vi "Tray_SetTray.vi"(7 "Initial color":u32(colorbox)=16448250, 8 "error in (no error)":errorcluster, 9 "GridSize":cluster{"x":u32, "y":u32}, 10 "MaxArea":cluster{"x":u32, "y":u32}, 11 "Tray in":refnum<vi>) -> (0 "error out":errorcluster)   [LabVIEW 2019]
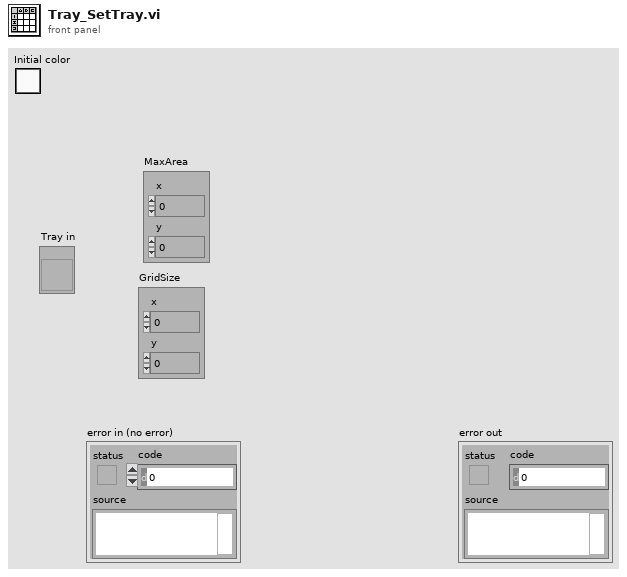
[diagram p1: front panel]
types:
  T1 = typedef "LVPositionTypeDef.ctl" = cluster{"Left":i32, "Top":i32}
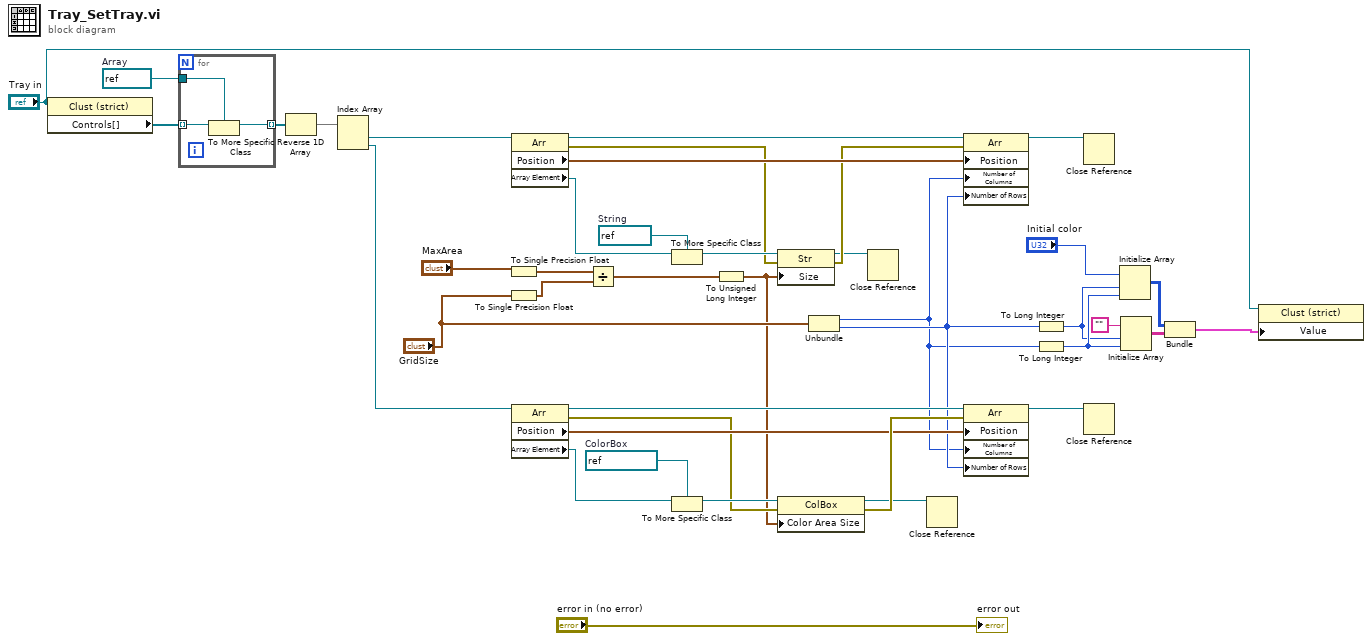
[diagram p0: block diagram]
diagram:
  w17 = refnum<vi> refnum  # Array
  w41 = refnum<vi> refnum  # String
  w38 = refnum<vi> refnum  # ColorBox
  n1 = property class="Clust (strict)"(reference="Tray in") -> ("Controls[]"=w18:refnum<vi>[])  [unwired: 1 in, 2 out]
  n2 = for {
    tunnel: w18 -> [w44] mode=indexing
    tunnel: w17 -> [w43]
    tunnel: [w42] -> w16 mode=indexing
    n3 = To More Specific Class(target class=w43, reference=w44) -> (specific class reference=w42:refnum<vi>)  [unwired: 1 in, 1 out]
  }
  n4 = Reverse 1D Array(array=w16) -> (reversed array=w15:refnum<vi>[])
  n5 = Index Array(array=w15) -> (element #1=w14:refnum<vi>, element #2=w13:refnum<vi>)  [unwired: 2 in]
  n6 = To Single Precision Float(number="MaxArea") -> (single precision float=w12:cluster{"x":sgl, "y":sgl})
  n7 = To Single Precision Float(number="GridSize") -> (single precision float=w10:cluster{"x":sgl, "y":sgl})
  n8 = property class="Arr"(reference=w14) -> (reference out=w32:refnum<vi>, error out=w33:errorcluster, "Position"=w35:T1, "Array Element"=w39:refnum<vi>)  [unwired: 1 in]
  n9 = property class="Arr"(reference=w13) -> (reference out=w29:refnum<vi>, error out=w28:errorcluster, "Position"=w30:T1, "Array Element"=w36:refnum<vi>)  [unwired: 1 in]
  n10 = Divide(x=w12, y=w10) -> (x/y=w27:cluster{"x":sgl, "y":sgl})
  n11 = To More Specific Class(target class=w41, reference=w39) -> (specific class reference=w40:refnum<vi>)  [unwired: 1 in, 1 out]
  n12 = To More Specific Class(target class=w38, reference=w36) -> (specific class reference=w37:refnum<vi>)  [unwired: 1 in, 1 out]
  n13 = To Unsigned Long Integer(number=w27) -> (unsigned 32bit integer=w9:cluster{"x":u32, "y":u32})
  n14 = property class="Str"(reference=w40, error in=w33, "Size"=w9) -> (reference out=w5:refnum<vi>, error out=w34:errorcluster)
  n15 = property class="ColBox"(reference=w37, error in=w28, "Color Area Size"=w9) -> (reference out=w8:refnum<vi>, error out=w31:errorcluster)
  n16 = Unbundle("GridSize") -> ("x"=w19:u32, "y"=w20:u32)
  n17 = Close Reference(reference=w5) -> ()  [unwired: 1 in, 1 out]
  n18 = Close Reference(reference=w8) -> ()  [unwired: 1 in, 1 out]
  n19 = property class="Arr"(reference=w32, error in=w34, "Position"=w35, "Number of Columns"=w19, "Number of Rows"=w20) -> (reference out=w6:refnum<vi>)  [unwired: 1 out]
  n20 = property class="Arr"(reference=w29, error in=w31, "Position"=w30, "Number of Columns"=w19, "Number of Rows"=w20) -> (reference out=w7:refnum<vi>)  [unwired: 1 out]
  n21 = To Long Integer(number=w20) -> (32bit integer=w23:i32)
  n22 = To Long Integer(number=w19) -> (32bit integer=w24:i32)
  n23 = Close Reference(reference=w6) -> ()  [unwired: 1 in, 1 out]
  n24 = Close Reference(reference=w7) -> ()  [unwired: 1 in, 1 out]
  n25 = Initialize Array("Initial color", w23, w24) -> (w25:u32[][])
  n26 = Initialize Array("" ("String"), w23, w24) -> (w26:string[][])
  n27 = Bundle(w25, w26) -> (w1:cluster{u32[][], string[][]})  [unwired: 1 in]
  n28 = property class="Clust (strict)"(reference="Tray in", "Value"=w1) -> ()  [unwired: 1 in, 2 out]
  "error out" <- "error in (no error)"
